vi "TPKT - Add Header.vi"(8 "error in (no error)":errorcluster, 10 "TPDU":T1 format="0x%02x") -> (0 "error out":errorcluster, 2 "TPKT":T1 format="0x%02x")   [LabVIEW 2014, in "S7NetCom.lvclass"]
doc: "Adds the 4-byte TPKT header to the TPDU.\n\n_____\nCopyright (c) 2019 Hampel Software Engineering (HSE), released under BSD license. More info can be found on https://dokuwiki.hampel-soft.com/code/hse/s7netcom. Original code published by Marc Christenson, Sisu Devices."
uses:
  S7NetCom.lvclass
  Controls/S7NetCom_HexByteArray.ctl
  Controls/S7NetCom_HexByte.ctl
panel:
  # "More info on https://dokuwiki.hampel-soft.com/code/hse/s7netcom\n\nCopyright (c) 2019, HAMPEL SOFTWARE ENGINEERING (HSE)\nOriginal code developed by Marc Christenson, Sisu Devices\nAll rights reserved.\n\nRedistribution and use in source and binary forms, with or without\nmodification, are permitted provided that the following conditions are met:\n\n1. Redistributions of source code must retain the above copyright\n   notice, this list of conditions and the following disclaimer.\n\n2. Redistributions in binary form must reproduce the above copyright\n   notice, this list of conditions and the following disclaimer in the\n   documentation and/or other materials provided with the distribution.\n\n3. All advertising materials mentioning features or use of this software\n   must display the following acknowledgement:\n   This product includes software developed by HAMPEL SOFTWARE ENGINEERING.\n\n4. Neither the name of HAMPEL SOFTWARE ENGINEERING nor the\n   names of its contributors may be used to endorse or promote products\n   derived from this software without specific prior written permission.\n\nTHIS SOFTWARE IS PROVIDED BY HAMPEL SOFTWARE ENGINEERING ''AS IS'' AND ANY\nEXPRESS OR IMPLIED WARRANTIES, INCLUDING, BUT NOT LIMITED TO, THE IMPLIED\nWARRANTIES OF MERCHANTABILITY AND FITNESS FOR A PARTICULAR PURPOSE ARE\nDISCLAIMED. IN NO EVENT SHALL HAMPEL SOFTWARE ENGINEERING BE LIABLE FOR ANY\nDIRECT, INDIRECT, INCIDENTAL, SPECIAL, EXEMPLARY, OR CONSEQUENTIAL DAMAGES\n(INCLUDING, BUT NOT LIMITED TO, PROCUREMENT OF SUBSTITUTE GOODS OR SERVICES;\nLOSS OF USE, DATA, OR PROFITS; OR BUSINESS INTERRUPTION) HOWEVER CAUSED AND\nON ANY THEORY OF LIABILITY, WHETHER IN CONTRACT, STRICT LIABILITY, OR TORT\n(INCLUDING NEGLIGENCE OR OTHERWISE) ARISING IN ANY WAY OUT OF THE USE OF THIS\nSOFTWARE, EVEN IF ADVISED OF THE POSSIBILITY OF SUCH DAMAGE."
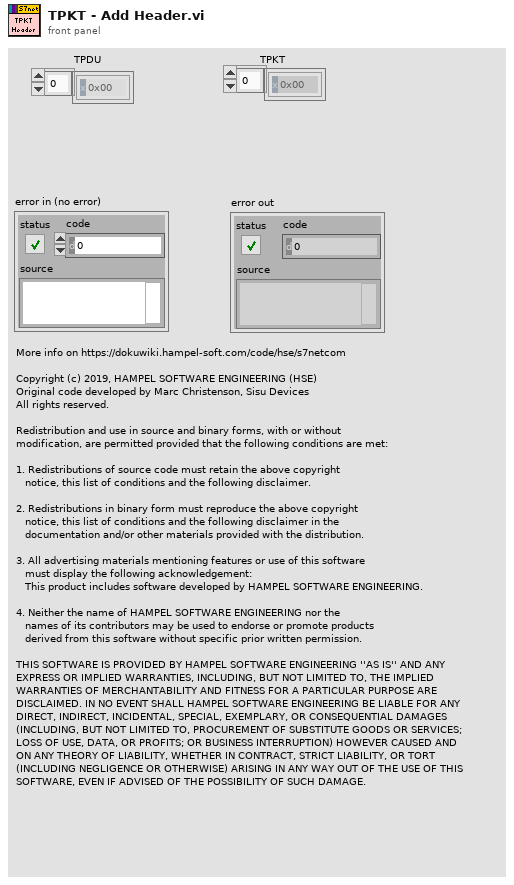
[diagram p1: front panel]
types:
  T1 = typedef "S7NetCom.lvclass/S7NetCom_HexByteArray.ctl" = T2[]
  T2 = typedef "S7NetCom.lvclass/S7NetCom_HexByte.ctl" = u8
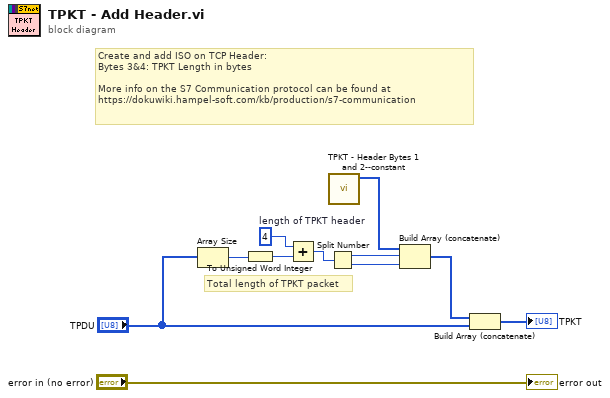
[diagram p0: block diagram]
diagram:
  w6 = u16 4  # length of TPKT header
  # "Total length of TPKT packet"
  # "Create and add ISO on TCP Header:\nBytes 3&4: TPKT Length in bytes\n\nMore info on the S7 Communication protocol can be found at\nhttps://dokuwiki.hampel-soft.com/kb/production/s7-communication"
  n1 = Array Size(array="TPDU") -> (size(s)=w4:i32)
  n2 = To Unsigned Word Integer(number=w4) -> (unsigned 16bit integer=w5:u16)
  n3 = Add(x=w6, y=w5) -> (x+y=w9:u16)
  n4 = Split Number(x=w9) -> (hi(x)=w8:u8, lo(x)=w7:u8)
  n5 = call "TPKT - Header Bytes 1 and 2--constant.vi"() -> ("TPKT Header Bytes 1 & 2"=w1:T2[])  [unwired: 11 in]
  n6 = Build Array (concatenate)(w1, w8, w7) -> (w2:T2[])
  n7 = Build Array (concatenate)(w2, "TPDU") -> (→"TPKT":T1)
  "error out" <- "error in (no error)"
